vi "OverlayInfo1.vi"(6 "Offset":sgl, 8 "Distance Points":cluster{"X":sgl, "Y":sgl}[](array[cluster]) {"Y" format="%.2f"; "X" format="%.2f"}, 9 "TotalDistance":sgl, 10 "Edges Coordinates in":cluster{"X":sgl, "Y":sgl}[](array[cluster]), 11 "Image in":T2) -> (0 "Oil Value":sgl, 1 "Water Value":sgl, 3 "Image Out":T2)   [LabVIEW 2012]
uses:
  <vilib>/vision/Image Controls.llb/IMAQ Image.ctl
panel:
  in  "Font, Size & Style":T1={"Desired Font (Application)"=enum."Application Font", "[User-specified Font]"={"Font Name"="", "Size"=72, "Strikeout?"=FALSE, "Italic?"=FALSE, "Underline?"=FALSE, "Outline?"=FALSE, "Shadow?"=FALSE, "Bold?"=TRUE, "Rotation Angle"=0.0}, "Horizontal Alignment"=0, "Vertical Alignment"=0} {"Vertical Alignment" items=["Bottom", "Top", "Baseline"]; "Horizontal Alignment" items=["Left", "Center", "Right"]; "[User-specified Font]"."Rotation Angle" format="%.2f"}
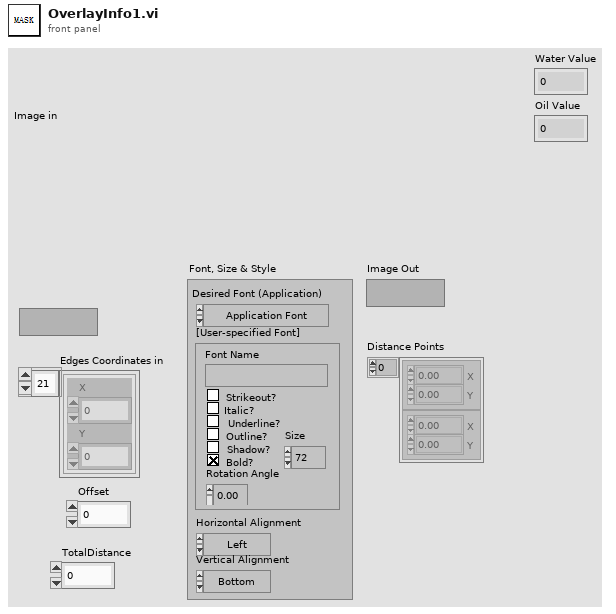
[diagram p1: front panel]
types:
  T1 = cluster{"Desired Font (Application)":enum16{"User-specified Font", "Application Font", "System Font", "Dialog Font"}, "[User-specified Font]":cluster{"Font Name":string, "Size":i16, "Strikeout?":bool, "Italic?":bool, "Underline?":bool, "Outline?":bool, "Shadow?":bool, "Bold?":bool, "Rotation Angle":dbl}, "Horizontal Alignment":i16, "Vertical Alignment":i16}
  T2 = typedef "IMAQ Image.ctl" = refnum<image>
  T3 = cluster{"Left":i32, "Top":i32, "Right":i32, "Bottom":i32}
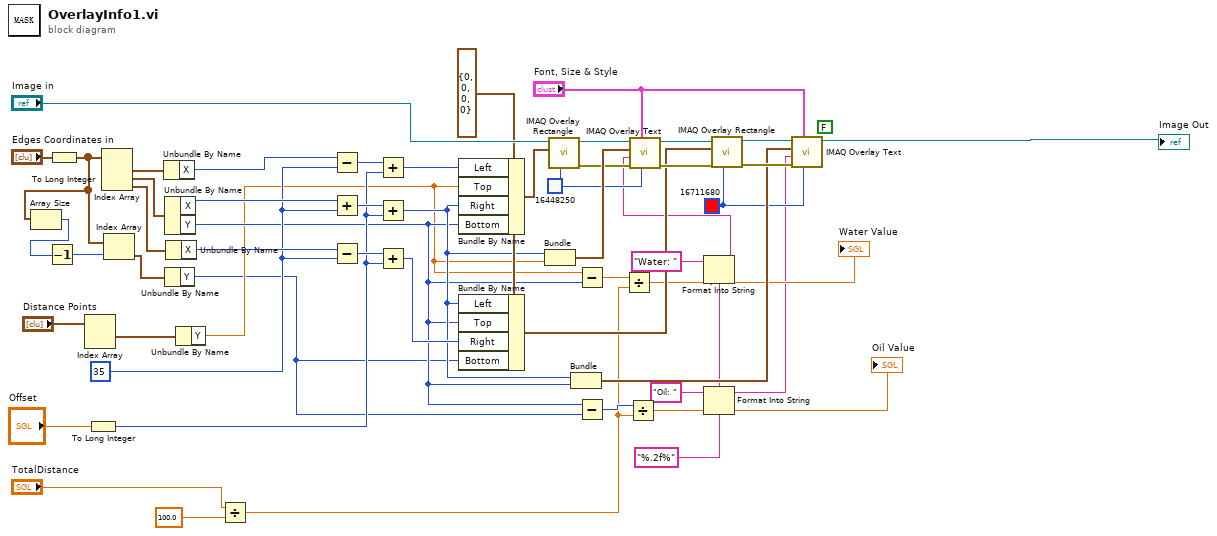
[diagram p0: block diagram]
diagram:
  (unwired) FALSE
  w16 = "%.2f%" ("format string")
  w31 = u32 16711680 ("Color")
  w32 = u32 16448250 ("Color")
  w27 = 35 ("y")
  n1 = To Long Integer(number="Edges Coordinates in") -> (32bit integer=w1:cluster{"X":i32, "Y":i32}[])
  n2 = Array Size(array=w1) -> (size(s)=w5:i32)
  n3 = Decrement(x=w5) -> (x-1=w4:i32)
  n4 = Index Array(array="Distance Points") -> (element #1=w8:cluster{"X":sgl, "Y":sgl})  [unwired: 2 in, 1 out]
  n5 = To Long Integer(number="Offset") -> (32bit integer=w11:i32)
  n6 = Index Array(array=w1) -> (element #1=w45:cluster{"X":i32, "Y":i32}, element #2=w46:cluster{"X":i32, "Y":i32}, element #3=w37:cluster{"X":i32, "Y":i32})  [unwired: 3 in]
  n7 = Index Array(array=w1, index=w4) -> (element=w3:cluster{"X":i32, "Y":i32})
  n8 = Unbundle By Name(w45) -> ("X"=w47:i32)
  n9 = Unbundle By Name(w46) -> ("X"=w48:i32, "Y"=w10:i32)
  n10 = Unbundle By Name(w3) -> ("Y"=w2:i32)
  n11 = Unbundle By Name(w37) -> ("X"=w36:i32)
  n12 = Unbundle By Name(w8) -> ("Y"=w7:sgl)
  n13 = Divide(x="TotalDistance", y=sgl 100.0) -> (x/y=w13:sgl)
  n14 = Subtract(x=w47, y=w27) -> (x-y=w50:i32)
  n15 = Add(x=w48, y=w27) -> (x+y=w51:i32)
  n16 = Subtract(x=w36, y=w27) -> (x-y=w35:i32)
  n17 = Add(x=w50, y=w11) -> (x+y=w44:i32)
  n18 = Add(x=w51, y=w11) -> (x+y=w24:i32)
  n19 = Add(x=w35, y=w11) -> (x+y=w28:i32)
  n20 = Bundle By Name(cluster=T3 {"Left"=0, "Top"=0, "Right"=0, "Bottom"=0} ("Rectangle"), "Left"=w44, "Top"=w7, "Right"=w24, "Bottom"=w10) -> (w29:T3)
  n21 = Bundle By Name(cluster=w29, "Left"=w24, "Top"=w10, "Right"=w28, "Bottom"=w2) -> (w34:T3)
  n22 = Bundle(w24, "Y"=w7) -> (w43:cluster{i32, "Y":sgl})  [unwired: 1 in]
  n23 = call "IMAQ Overlay Rectangle"("Color"=w32, "Rectangle"=w29, "Image"="Image in") -> ("error out"=w40:errorcluster, "Image Out"=w53:T2)  [unwired: 7 in]
  n24 = Bundle(w24, "Y"=w10) -> (w33:cluster{i32, "Y":i32})  [unwired: 1 in]
  n25 = Subtract(x=w7, y=w10) -> (x-y=w23:sgl)
  n26 = Subtract(x=w10, y=w2) -> (x-y=w22:i32)
  n27 = Divide(x=w23, y=w13) -> (x/y=w21:sgl)
  "Water Value" <- w21
  n28 = Divide(x=w22, y=w13) -> (x/y=w17:sgl)
  "Oil Value" <- w17
  n29 = Format Into String(format string=w16, initial string="Water: ", w21) -> (resulting string=w19:string)  [unwired: 1 in, 1 out]
  n30 = call "IMAQ Overlay Text"("Text Color (black)"=w32, "Font, Size & Style"="Font, Size & Style", "error in (no error)"=w40, "String"=w19, "Origin"=w43, "Image"=w53) -> ("error out"=w39:errorcluster, "Image Out"=w41:T2)  [unwired: 4 in]
  n31 = Format Into String(format string=w16, initial string="Oil: ", w17) -> (resulting string=w15:string)  [unwired: 1 in, 1 out]
  n32 = call "IMAQ Overlay Rectangle"("Color"=w31, "error in (no error)"=w39, "Rectangle"=w34, "Image"=w41) -> ("error out"=w38:errorcluster, "Image Out"=w42:T2)  [unwired: 6 in]
  n33 = call "IMAQ Overlay Text"("Text Color (black)"=w31, "Font, Size & Style"="Font, Size & Style", "error in (no error)"=w38, "String"=w15, "Origin"=w33, "Image"=w42) -> ("Image Out"=→"Image Out":T2)  [unwired: 4 in, 1 out]
